vi "Write Color Area Size Height.vi"(8 "error in (no error)":errorcluster, 10 "Height":u32, 11 "ColorRamp.lvclass in":refnum<class "ColorRamp.lvclass">) -> (0 "error out":errorcluster, 3 "ColorRamp.lvclass out":refnum<class "ColorRamp.lvclass">)   [LabVIEW 2015, in "ColorRamp.lvclass"]
uses:
  ColorRamp.lvclass
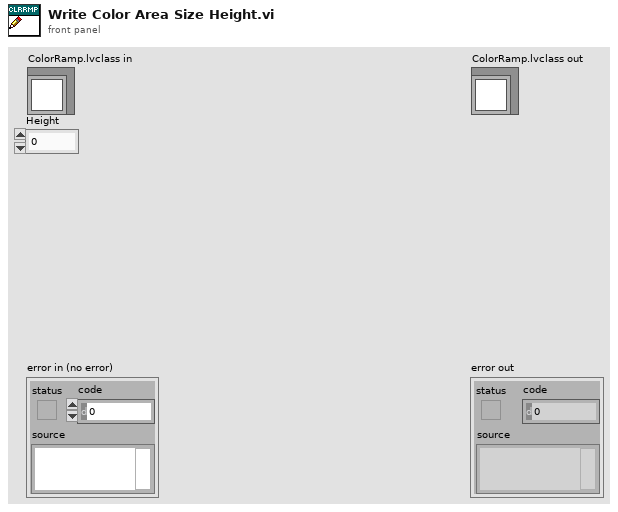
[diagram p1: front panel]
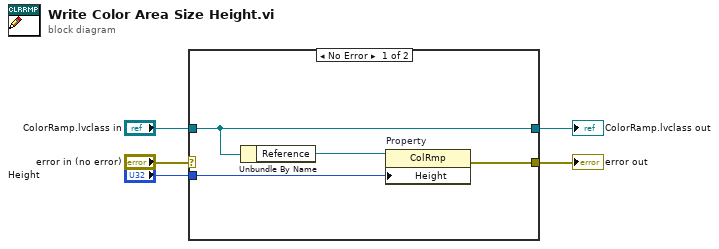
[diagram p0: block diagram]
diagram:
  n1 = case shown="No Error" "error in (no error)" {
    selector: "error in (no error)" -> [_ w11]
    tunnel: [w9 w11] -> w4
    tunnel: [w7 w10] -> w2
    tunnel: "ColorRamp.lvclass in" -> [w7 w10]
    tunnel: "Height" -> [w8 _]
    frame No Error {
      n2 = Unbundle By Name(w7) -> ("Reference"=w6:refnum<vi>)
      n3 = property on="Property" class="ColRmp"(reference=w6, "Height"=w8) -> (error out=w9:errorcluster)  [unwired: 1 in, 1 out]
    }
    frame Error {
    }
  }
  "error out" <- w4
  "ColorRamp.lvclass out" <- w2
